vi "Read VISA resource name.vi"(8 "error in (no error)":errorcluster, 11 "Agilent 34401a in":refnum<class "Agilent 34401a.lvclass">) -> (0 "error out":errorcluster, 2 "VISA resource name":refnum<visa-resource-name>, 3 "Agilent 34401a out":refnum<class "Agilent 34401a.lvclass">)   [LabVIEW 2013, in "Agilent 34401a.lvclass"]
uses:
  Agilent 34401a.lvclass
  Agilent 34401a.lvclass/Agilent 34401a.ctl
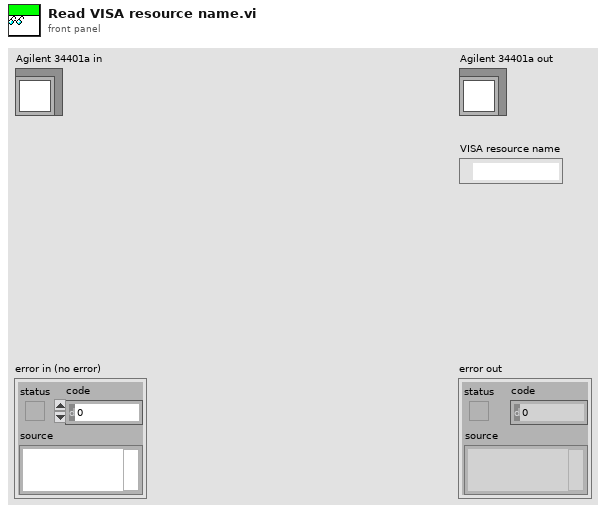
[diagram p1: front panel]
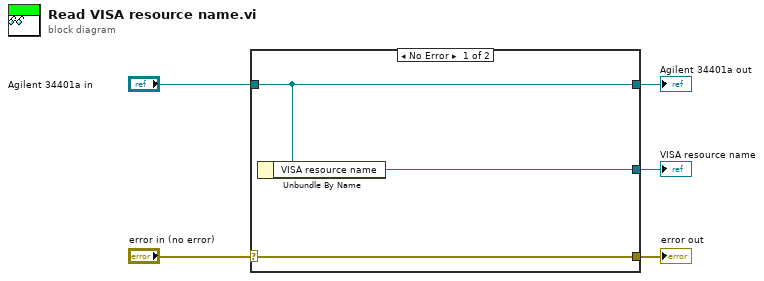
[diagram p0: block diagram]
diagram:
  n1 = case shown="No Error" "error in (no error)" {
    selector: "error in (no error)" -> [w8 w9]
    tunnel: [w8 w9] -> w4
    tunnel: [w7 w10] -> w2
    tunnel: "Agilent 34401a in" -> [w7 w10]
    tunnel: [w6 _] -> w1
    frame No Error {
      n2 = Unbundle By Name(w7) -> ("VISA resource name"=w6:refnum<visa-resource-name>)
    }
    frame Error {
    }
  }
  "error out" <- w4
  "Agilent 34401a out" <- w2
  "VISA resource name" <- w1
